vi "Tension Viewer.vi"() -> ()   [LabVIEW 2021]
panel:
  in  "R":dbl=0.5
  in  "Samples":i32=128
  out "Waveform Chart":T1(graph)={"Tension[0]"=45.42905638821776, "Tension[1]"=32.07310109333792, "Tension[2]"=50.46553411279194, "Tension[3]"=0.0, "Tension[4]"=0.0, "Tension[5]"=0.0, "Tension[6]"=0.0, "Tension[7]"=0.0, "Tension[8]"=0.0}
  in  "Total Time":dbl=10.0 format="%#_13g"
  out "XY Graph":cluster{dbl[], dbl[]}[](graph)=[{[-0.3019938329609982], [-0.3890188411994382]}, {[0.0, 0.0, 0.0, 0.0, 0.0, 0.0, 0.0, 0.0, 0.0, 0.0, 0.0, 0.0, 0.0, 0.0, 0.0, 0.0, 0.0, 0.0, 0.0, 0.0, 0.0, 0.0, 0.0, 0.0, 0.0, 0.0, 0.0, 0.0, 0.0, 0.0, 0.0, 0.0, 0.0, -0.0, -0.0, -0.0, -0.0, -0.0, -0.0, -0.0, -0.0, -0.0, -0.0, -0.0, -0.0, -0.0, -0.0, -0.0, -0.0, -0.0, -0.0, -0.0, -0.0, -0.0, -0.0, -0.0, -0.0, -0.0, -0.0, -0.0, -0.0, -0.0, -0.0, -0.0, -0.0, -0.0, -0.0, -0.0, -0.0, -0.0, -0.0, -0.0, -0.0, -0.0, -0.0, -0.0, -0.0, -0.0, -0.0, -0.0, -0.0, -0.0, -0.0, -0.0, -0.0, -0.0, -0.0, -0.0, -0.0, -0.0, -0.0, -0.0, -0.0, -0.0, -0.0, -0.0, -0.0, 0.0, 0.0, 0.0, 0.0, 0.0, 0.0, 0.0, 0.0, 0.0, 0.0, 0.0, 0.0, 0.0, 0.0, 0.0, 0.0, 0.0, 0.0, 0.0, 0.0, 0.0, 0.0, 0.0, 0.0, 0.0, 0.0, 0.0, 0.0, 0.0, 0.0, 0.0], [0.0, 0.0, 0.0, 0.0, 0.0, 0.0, 0.0, 0.0, 0.0, 0.0, 0.0, 0.0, 0.0, 0.0, 0.0, 0.0, 0.0, 0.0, 0.0, 0.0, 0.0, 0.0, 0.0, 0.0, 0.0, 0.0, 0.0, 0.0, 0.0, 0.0, 0.0, 0.0, 0.0, 0.0, 0.0, 0.0, 0.0, 0.0, 0.0, 0.0, 0.0, 0.0, 0.0, 0.0, 0.0, 0.0, 0.0, 0.0, 0.0, 0.0, 0.0, 0.0, 0.0, 0.0, 0.0, 0.0, 0.0, 0.0, 0.0, 0.0, 0.0, 0.0, 0.0, 0.0, 0.0, -0.0, -0.0, -0.0, -0.0, -0.0, -0.0, -0.0, -0.0, -0.0, -0.0, -0.0, -0.0, -0.0, -0.0, -0.0, -0.0, -0.0, -0.0, -0.0, -0.0, -0.0, -0.0, -0.0, -0.0, -0.0, -0.0, -0.0, -0.0, -0.0, -0.0, -0.0, -0.0, -0.0, -0.0, -0.0, -0.0, -0.0, -0.0, -0.0, -0.0, -0.0, -0.0, -0.0, -0.0, -0.0, -0.0, -0.0, -0.0, -0.0, -0.0, -0.0, -0.0, -0.0, -0.0, -0.0, -0.0, -0.0, -0.0, -0.0, -0.0, -0.0, -0.0, -0.0]}]
  out "Cluster":T2={"Time"=6.9, "X"=-0.3019938329609982, "Y"=-0.3890188411994382, "Tension"=[45.42905638821776, 32.07310109333792, 50.46553411279194]}
  out "String":string="Init Done!"
  in  "stop 2":bool
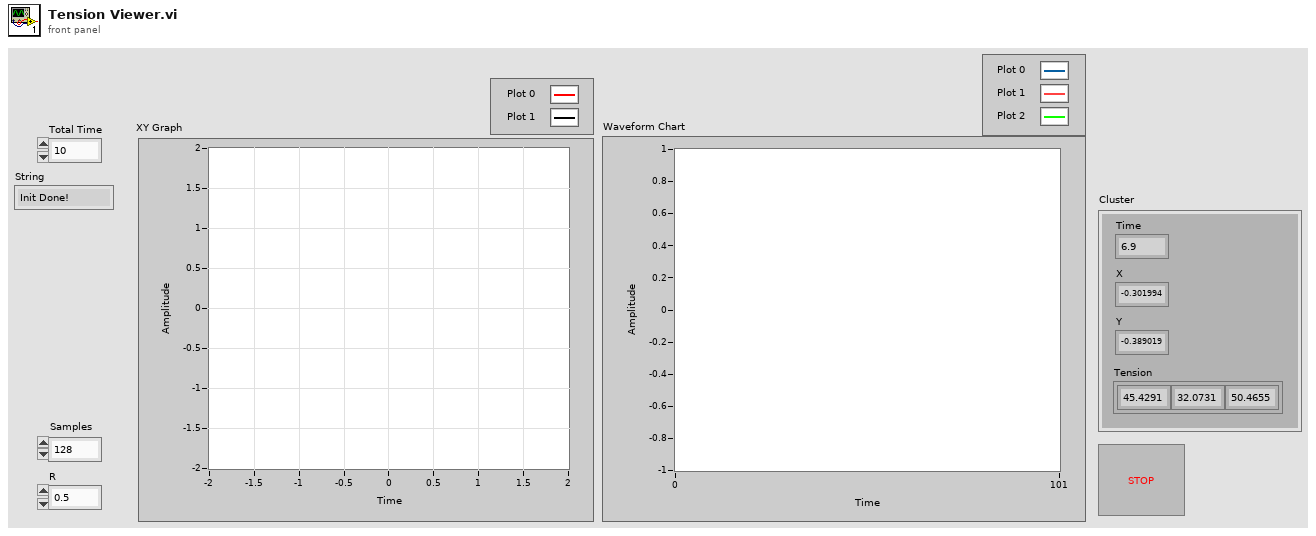
[diagram p1: front panel]
types:
  T1 = cluster{"Tension[0]":dbl, "Tension[1]":dbl, "Tension[2]":dbl, "Tension[3]":dbl, "Tension[4]":dbl, "Tension[5]":dbl, "Tension[6]":dbl, "Tension[7]":dbl, "Tension[8]":dbl}
  T2 = cluster{"Time":dbl, "X":dbl, "Y":dbl, "Tension":dbl[]}
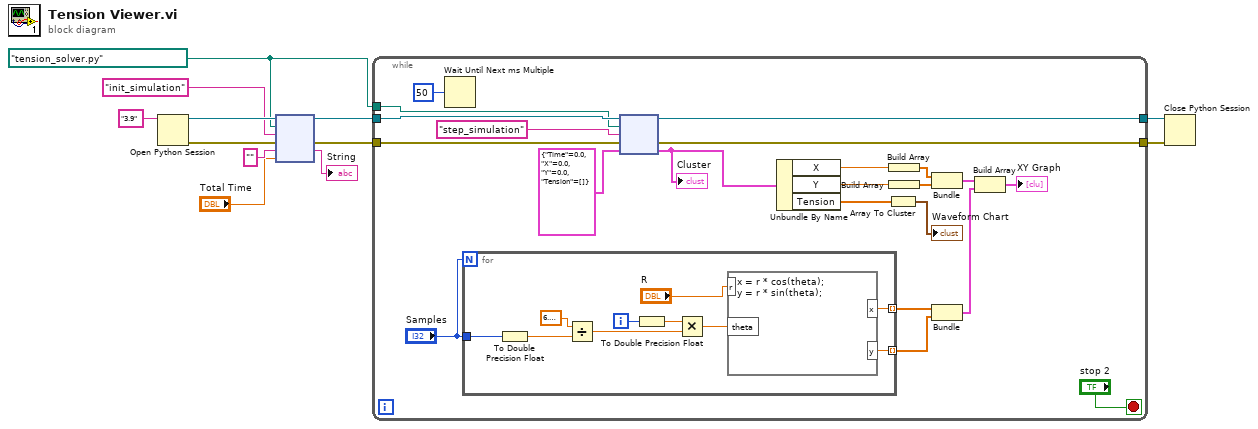
[diagram p0: block diagram]
diagram:
  w5 = path "tension_solver.py" ("module path")
  n1 = Open Python Session(python version="3.9" ("Python version")) -> (session out=w11:refnum<k35>, error out=w9:errorcluster)  [unwired: 2 in]
  n2 = node(w11, w5, "init_simulation" ("function name"), w9, "" ("String 2"), "Total Time") -> (w8:refnum<k35>, w6:errorcluster, →"String":string)  [unwired: 1 in, 2 out]
  n3 = while {
    tunnel: w8 -> [w28]
    tunnel: [w31] -> w7
    tunnel: w6 -> [w30]
    tunnel: [w29] -> w1
    tunnel: w5 -> [w27]
    stop <- "stop 2" stop-if-true
    n4 = Wait Until Next ms Multiple(millisecond multiple=u32 50) -> ()  [unwired: 1 out]
    n5 = for {
      N: "Samples" -> [_]
      tunnel: [w44] -> w21 mode=indexing
      tunnel: [w43] -> w20 mode=indexing
      tunnel: "Samples" -> [w38]
      i -> [w39]
      n6 = To Double Precision Float(number=w38) -> (double precision float=w36:dbl)
      n7 = Divide(x=6.283185307179586, y=w36) -> (x/y=w41:dbl)
      n8 = To Double Precision Float(number=w39) -> (double precision float=w37:dbl)
      n9 = Multiply(x=w37, y=w41) -> (x*y=w40:dbl)
      n10 = formula code="x = r * cos(theta);\ny = r * sin(theta);"("r"="R", "theta"=w40) -> ("x"=w44:dbl, "y"=w43:dbl)
    }
    n11 = node(w28, w27, "step_simulation" ("function name"), w30, T2 {"Time"=0.0, "X"=0.0, "Y"=0.0, "Tension"=[]} ("Cluster")) -> (w31:refnum<k35>, w29:errorcluster, w26:T2)  [unwired: 2 out]
    "Cluster" <- w26
    n12 = Unbundle By Name(w26) -> ("X"=w16:dbl, "Y"=w15:dbl, "Tension"=w23:dbl[])
    n13 = Array To Cluster(array=w23) -> (cluster=→"Waveform Chart":T1)
    n14 = Build Array(w16) -> (w13:dbl[])
    n15 = Build Array(w15) -> (w14:dbl[])
    n16 = Bundle(w13, w14) -> (w17:cluster{dbl[], dbl[]})  [unwired: 1 in]
    n17 = Bundle(w21, w20) -> (w19:cluster{dbl[], dbl[]})  [unwired: 1 in]
    n18 = Build Array(w17, w19) -> (→"XY Graph":cluster{dbl[], dbl[]}[])
  }
  n19 = Close Python Session(session in=w7, error in=w1) -> ()  [unwired: 1 out]
